vi "LuaVIEW Preprocessor.vi"(0 "path":path, 1 "parent index":i32, 5 "task info in":T2 {"handle mask" format="%.0b"; "allow mask" format="%.0b"; "signal flags" format="%.0b"}, 7 "script":string, 9 "main path valid?":bool, 11 "error in (no error)":errorcluster, 12 "main script?":bool, 13 "swap? (false)":bool) -> (4 "import paths":path[](array[path]), 6 "task info out":T2 {"handle mask" format="%.0b"; "allow mask" format="%.0b"; "signal flags" format="%.0b"}, 8 "script info":T1, 15 "error out":errorcluster)   [LabVIEW 2012]
doc: "Extract task configuration keywords from a script and configure the task state."
uses:
  typedefs/clusters/LuaVIEW Task Info.ctl
  typedefs/t_LuaVIEW Task Modes.ctl
  typedefs/t_LuaVIEW Reference.ctl
  typedefs/clusters/LuaVIEW Script Info.ctl
  typedefs/t_LuaVIEW Task List Methods.ctl
  typedefs/et_LuaVIEW CIN Actions.ctl
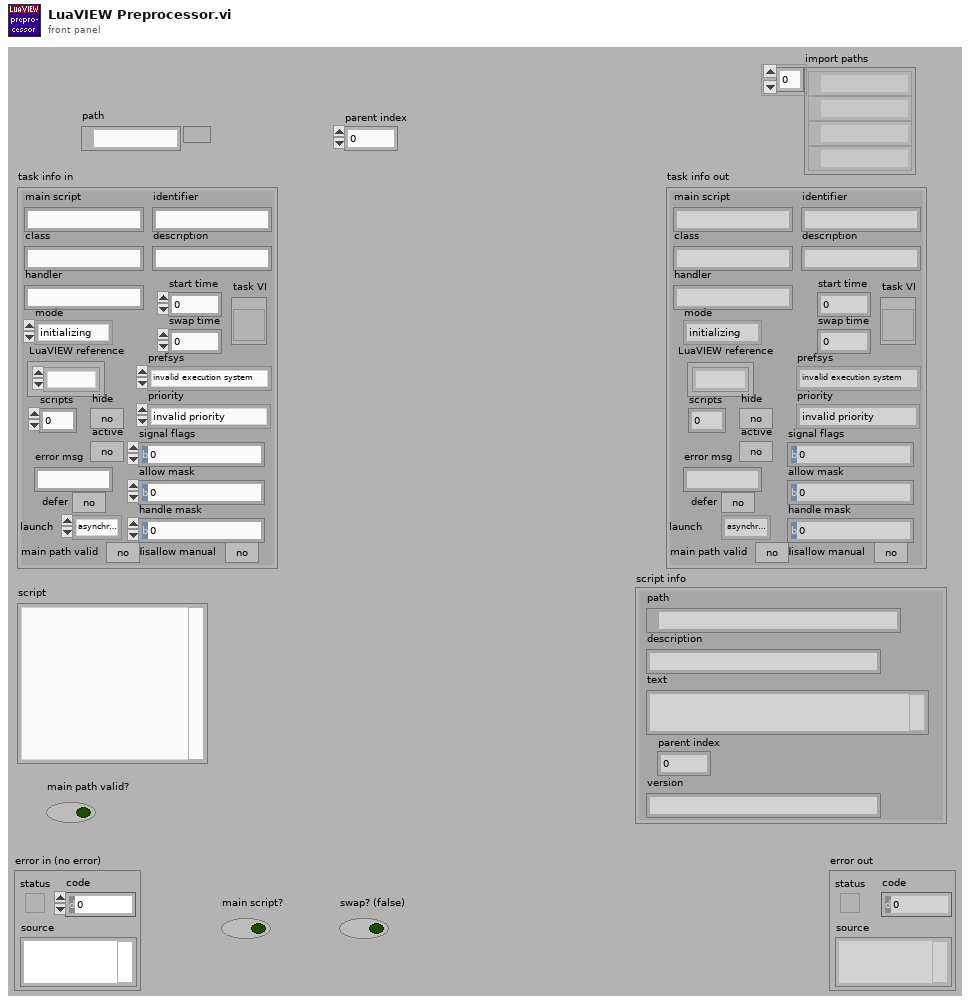
[diagram p1: front panel]
types:
  T1 = typedef "LuaVIEW Script Info.ctl" = cluster{"path":path, "description":string, "text":string, "parent index":i32, "version":string}
  T2 = typedef "LuaVIEW Task Info.ctl" = cluster{"main script":string, "identifier":string, "class":string, "description":string, "mode":T3, "handler":string, "LuaVIEW reference":T4, "scripts":i32, "hide":bool, "active":bool, "error msg":string, "defer":bool, "launch":enum16{"asynchronous", "manual", "synchronous"}, "main path valid":bool, "start time":dbl, "swap time":dbl, "task VI":refnum<vi>, "prefsys":enum32{"invalid execution system", "user interface", "standard", "instrument i/o", "data acquisition", "other 1", "other 2", "same as caller"}, "priority":enum32{"invalid priority", "background priority", "normal priority", "above normal priority", "high priority", "time critical priority", "subroutine"}, "signal flags":u32, "allow mask":u32, "handle mask":u32, "disallow manual":bool}
  T3 = typedef "t_LuaVIEW Task Modes.ctl" = enum16{"initializing", "running", "executing", "paused", "error", "swapping"}
  T4 = typedef "t_LuaVIEW Reference.ctl" = refnum<k1>
  T5 = typedef "t_LuaVIEW Task List Methods.ctl" = enum16{"clear list", "add", "test", "remove", "get ref", "get task info", "get list", "get script info", "ongoing?", "resume", "pause", "stop", "confirm", "message"}
  T6 = typedef "et_LuaVIEW CIN Actions.ctl" = enum16{"checksynopsis", "_open", "_registerpublic", "_registerexport", "__never_an_error_result_ns", "luaversion", "cinversion", "_totals", "_taskcount", "pathological", "_unregnextpublic", "registryusecount", "__per_state_actions", "regsetprivate", "regsetindex", "regsetmodule", "_revokeexports", "_usepublic", "prepare", "compile", "execute", "call", "unregstaterefs", "_close", "pullboolean", "pullnumber", "pullI8", "pullU8", "pullI16", "pullU16", "pullI32", "pullU32", "pullobject", "pullrefnum", "pullstring", "pullflat", "pushflat", "pushobject", "getattribute", "setattribute", "stacktostring", "_startyieldtest", "_endyieldtest", "_pollprintbuffer", "__never_an_error_result_ps", "_pollexport", "setclone", "forcecleanup", "gettop", "clearstack", "insert", "pushboolean", "pushnumber", "pushrefnum", "pushstring", "pushnil", "pushvalue", "gettaskref", "settaskref"}
  T7 = cluster{"line":i32, "keyword":string, "value":string}[]
  T8 = cluster{"line":i32, "keyword":string, "value":string}
  T9 = enum32{"invalid execution system", "user interface", "standard", "instrument i/o", "data acquisition", "other 1", "other 2", "same as caller"}
  T10 = enum32{"invalid priority", "background priority", "normal priority", "above normal priority", "high priority", "time critical priority", "subroutine"}
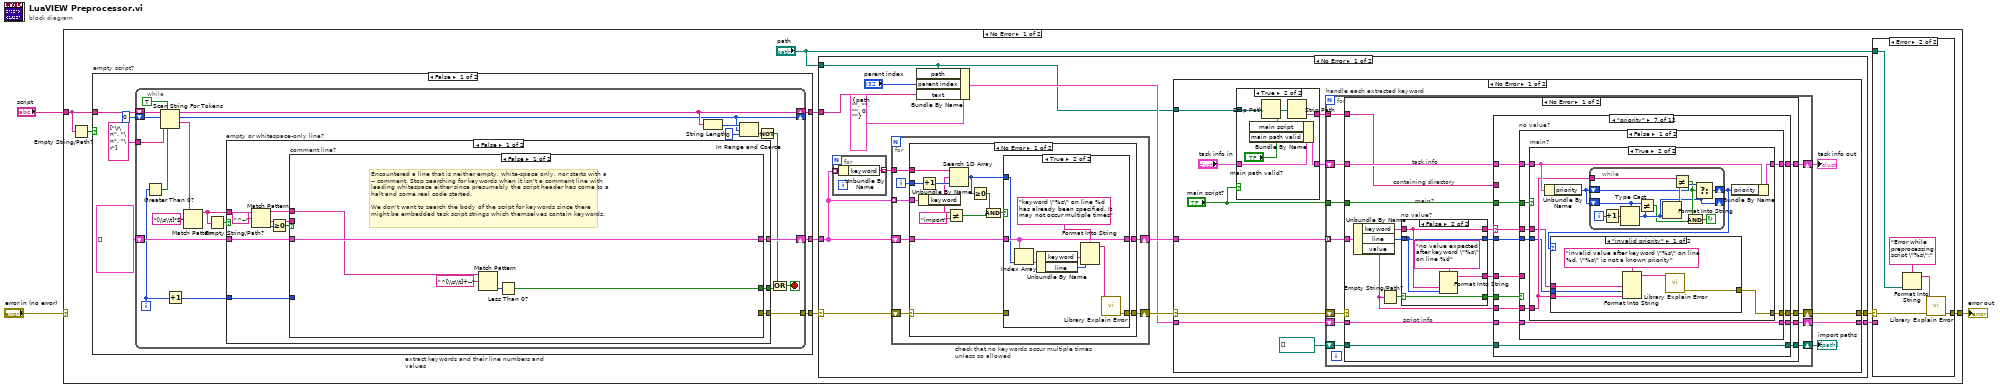
[diagram p0: block diagram]
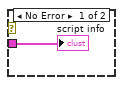
[diagram p2: hidden frame]
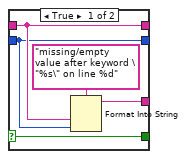
[diagram p4: hidden frame]
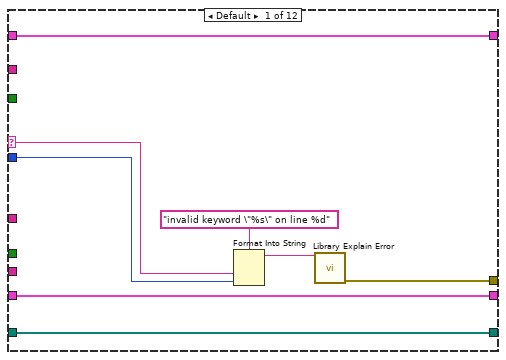
[diagram p5: hidden frame]
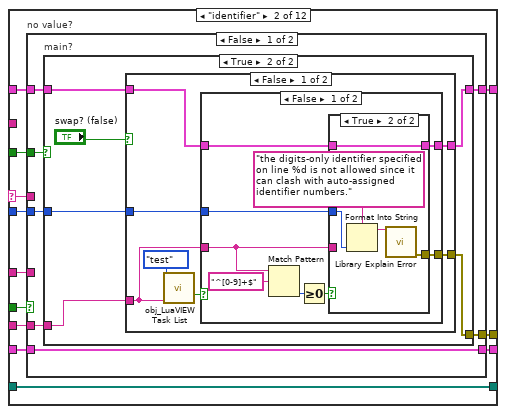
[diagram p6: hidden frame]
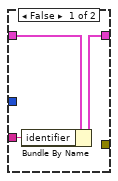
[diagram p8: hidden frame]
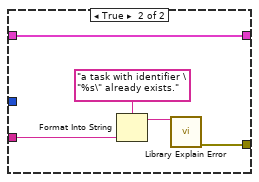
[diagram p9: hidden frame]
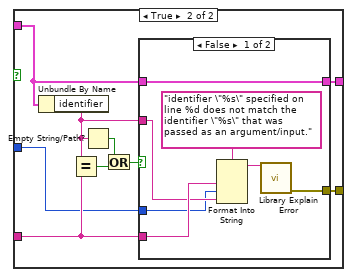
[diagram p10: hidden frame]
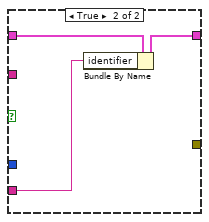
[diagram p11: hidden frame]
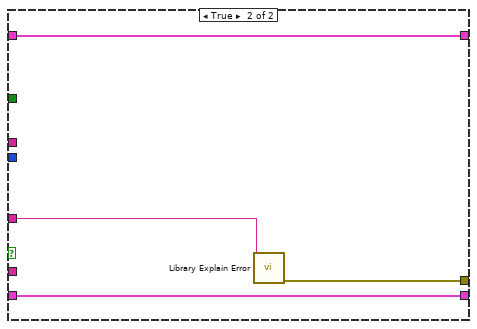
[diagram p12: hidden frame]
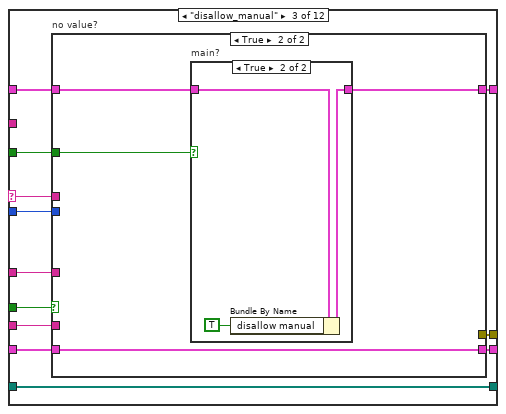
[diagram p13: hidden frame]
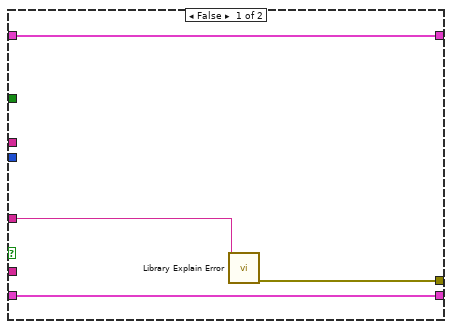
[diagram p14: hidden frame]
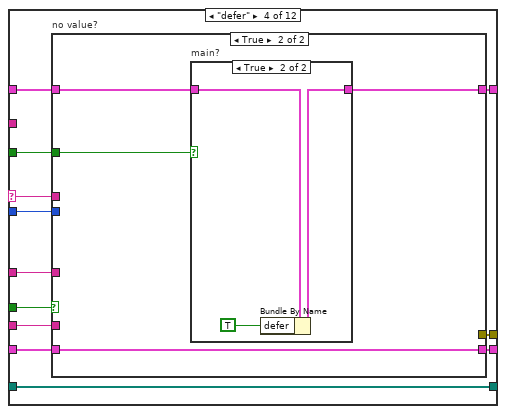
[diagram p16: hidden frame]
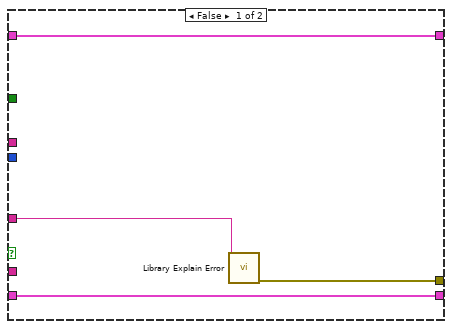
[diagram p17: hidden frame]
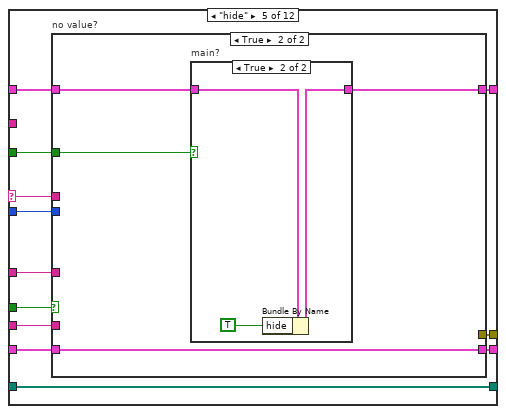
[diagram p19: hidden frame]
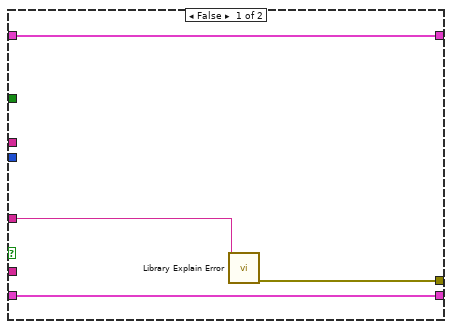
[diagram p20: hidden frame]
diagram:
  n1 = case shown="No Error" "error in (no error)" {
    selector: "error in (no error)" -> [_ w646]
    tunnel: "script" -> [w11 _]
    tunnel: [w5 w646] -> w1
    frame No Error {
      n2 = Empty String/Path?(string/path=w11) -> (empty?=w12:bool)
      n3 = case "empty script?" shown="False" w12 {
        tunnel: w11 -> [w539 w643]
        tunnel: [w537 w644] -> w10
        tunnel: [w536 w643] -> w9
        tunnel: [w535 _] -> w8
        frame False {
          n4 = while "extract keywords and their line numbers and values" {
            shift-right: [w547] -> w536
            shift-left: w539 -> [w563]
            tunnel: string[] ["\r\n", "\n", "\r"] ("delimiters (\\s,\\t,\\r,\\n)") -> [w562]
            shift-right: [w545] -> _
            shift-left: 0 ("offset past token") -> [w561]
            shift-right: [w548] -> w535
            shift-left: T7 [] -> [w554]
            tunnel: [w550] -> w537
            i -> [w551]
            stop <- w553 stop-if-true
            n5 = Greater Than 0?(x=w551) -> (x > 0?=w560:bool)
            n6 = Scan String For Tokens(4:w560, 5:TRUE ("allow empty tokens? (F)"), 6:w562, 8:w561, 9:w563) -> (1:w558:string, 2:w545:i32, 3:w547:string)  [unwired: 1 in, 1 out]
            n7 = Increment(x=w551) -> (x+1=w549:i32)
            n8 = Match Pattern(string=w558, regular expression="[\\s\\t]*$") -> (before substring=w556:string)  [unwired: 1 in, 3 out]
            n9 = Empty String/Path?(string/path=w556) -> (empty?=w555:bool)
            n10 = case "empty or whitespace-only line?" shown="False" w555 {
              tunnel: w556 -> [w573 _]
              tunnel: [w569 _] -> w552
              tunnel: w554 -> [w567 w642]
              tunnel: [w568 _] -> w550
              tunnel: w549 -> [w566 _]
              tunnel: [w565 w642] -> w548
              frame False {
                n11 = Match Pattern(string=w573, regular expression="^--") -> (before substring=w564:string, after substring=w570:string, offset past match=w572:i32)  [unwired: 1 in, 1 out]
                n12 = Greater Or Equal To 0?(x=w572) -> (x >= 0?=w571:bool)
                n13 = case "comment line?" shown="False" w571 {
                  tunnel: w570 -> [_ w580]
                  tunnel: [w576 w583] -> w569
                  tunnel: [_ w584] -> w568
                  tunnel: w567 -> [w579 w582]
                  tunnel: w566 -> [_ w585]
                  tunnel: [w579 w581] -> w565
                  tunnel: w564 -> [w575 _]
                  frame False {
                    # "Encountered a line that is neither empty, white-space only, nor starts with a -- comment. Stop searching for keywords when it isn't a comment line with leading whitespace either since presumably the script header has come to a halt and some real code started.\n\nWe don't want to search the body of the script for keywords since there might be embedded task script strings which themselves contain keywords."
                    n14 = Match Pattern(string=w575, regular expression="^[\\s\\t]+--") -> (offset past match=w577:i32)  [unwired: 1 in, 3 out]
                    n15 = Less Than 0?(x=w577) -> (x < 0?=w576:bool)
                  }
                  frame True {
                    n16 = Match Pattern(string=w580, regular expression="^#[a-z_]+") -> (match substring=w587:string, after substring=w588:string, offset past match=w592:i32)  [unwired: 1 in, 1 out]
                    n17 = Index Array(array=w582, index=-1) -> (element=w586:T8)
                    n18 = Greater Or Equal To 0?(x=w592) -> (x >= 0?=w590:bool)
                    n19 = case "looks like a keyword?" shown="True" w590 {
                      tunnel: w588 -> [_ w601]
                      tunnel: w587 -> [_ w606]
                      tunnel: w586 -> [_ w605]
                      tunnel: w585 -> [_ w604]
                      tunnel: [_ w594] -> w584
                      tunnel: [_ w595] -> w583
                      tunnel: w582 -> [w593 w598]
                      tunnel: [w593 w596] -> w581
                      frame False {
                      }
                      frame True {
                        n20 = String Subset(string=w606, offset (0)=1) -> (substring=w603:string)  [unwired: 1 in]
                        n21 = Bundle By Name(cluster=w605, "keyword"=w603, "line"=w604) -> (w599:T8)
                        n22 = Match Pattern(string=w601, regular expression="^[\\s\\t]*") -> (after substring=w597:string)  [unwired: 1 in, 3 out]
                        n23 = Empty String/Path?(string/path=w597) -> (empty?=w600:bool)
                        n24 = case "no trailing value?" shown="False" w600 {
                          tunnel: w599 -> [w613 w640]
                          tunnel: w598 -> [w614 w641]
                          tunnel: w597 -> [w625 _]
                          tunnel: [w612 w639] -> w596
                          tunnel: [w610 _] -> w595
                          tunnel: [w611 _] -> w594
                          frame False {
                            n25 = Search/Split String(string=w625, offset (0)=1) -> (substring before match=w619:string, match + rest of string=w622:string)  [unwired: 1 in, 1 out]
                            n26 = Equal?(x="\"" ("y"), y=w619) -> (x = y?=w617:bool)
                            n27 = String Length(string=w622) -> (length=w623:i32)
                            n28 = Decrement(x=w623) -> (x-1=w621:i32)
                            n29 = Search/Split String(string=w622, offset (0)=w621) -> (substring before match=w608:string, match + rest of string=w609:string)  [unwired: 1 in, 1 out]
                            n30 = Equal?(x="\"" ("y"), y=w609) -> (x = y?=w616:bool)
                            n31 = And(x=w617, y=w616) -> (x .and. y?=w615:bool)
                            n32 = case "proper double-quote delimited value?" shown="False" w615 {
                              tunnel: w614 -> [w633 w638]
                              tunnel: w613 -> [w632 w637]
                              tunnel: [w633 w635] -> w612
                              tunnel: [w631 _] -> w611
                              tunnel: [TRUE _] -> w610
                              tunnel: w608 -> [_ w634]
                              frame False {
                                n33 = Unbundle By Name(w632) -> ("keyword"=w628:string, "line"=w627:i32)
                                n34 = Format Into String(format string="value for keyword \"%s\" on line %d should be enclosed in double quotes.", w628, w627) -> (resulting string=w629:string)  [unwired: 2 in, 1 out]
                                n35 = call "Library Explain Error.vi"("explanation prefix (none)"=w629) -> ("explained error"=w631:errorcluster)  [unwired: 14 in]
                              }
                              frame True {
                                n36 = Bundle By Name(cluster=w637, "value"=w634) -> (w636:T8)
                                n37 = Build Array (concatenate)(w638, w636) -> (w635:T7)
                              }
                            }
                          }
                          frame True {
                            n38 = Build Array (concatenate)(w641, w640) -> (w639:T7)
                          }
                        }
                      }
                    }
                  }
                }
              }
              frame True {
              }
            }
            n39 = String Length(string=w547) -> (length=w546:i32)
            n40 = In Range and Coerce(upper limit=w546, x=w545, lower limit=0) -> (In Range?=w543:bool)  [unwired: 1 out]
            n41 = Not(x=w543) -> (.not. x?=w542:bool)
            n42 = Or(x=w542, y=w552) -> (x .or. y?=w553:bool)
          }
        }
        frame True {
          n43 = call "Library Explain Error.vi"("explanation prefix (none)"="script is empty") -> ("explained error"=w644:errorcluster)  [unwired: 14 in]
        }
      }
      n44 = case shown="No Error" w10 {
        selector: w10 -> [w30 w534]
        tunnel: w9 -> [w24 _]
        tunnel: w8 -> [w28 _]
        tunnel: "path" -> [w19 _]
        tunnel: [w21 _] -> w7
        tunnel: [w20 w534] -> w6
        frame No Error {
          n45 = for {
            tunnel: w28 -> [w533] mode=indexing
            tunnel: [w532] -> w29 mode=indexing
            n46 = Unbundle By Name(w533) -> ("keyword"=w532:string)
          }
          n47 = for "check that no keywords occur multiple times unless so allowed" {
            tunnel: w28 -> [w505] mode=indexing
            shift-right: [w499] -> w27
            shift-left: w30 -> [w503]
            tunnel: w29 -> [w502]
            shift-right: [w500] -> w26
            shift-left: w28 -> [w501]
            i -> [w504]
            n48 = case shown="No Error" w503 {
              selector: w503 -> [w506 w531]
              tunnel: w502 -> [w519 _]
              tunnel: w505 -> [w518 _]
              tunnel: w504 -> [w517 _]
              tunnel: w501 -> [w509 w530]
              tunnel: [w508 w530] -> w500
              tunnel: [w507 w531] -> w499
              frame No Error {
                n49 = Unbundle By Name(w518) -> ("keyword"=w515:string)
                n50 = Increment(x=w517) -> (x+1=w516:i32)
                n51 = Not Equal?(x=w515, y="import") -> (x != y?=w512:bool)
                n52 = Search 1D Array(1D array=w519, element=w515, start index (0)=w516) -> (index of element=w510:i32)
                n53 = Greater Or Equal To 0?(x=w510) -> (x >= 0?=w513:bool)
                n54 = And(x=w513, y=w512) -> (x .and. y?=w511:bool)
                n55 = case shown="True" w511 {
                  tunnel: w510 -> [_ w528]
                  tunnel: w509 -> [w520 w529]
                  tunnel: [w520 w529] -> w508
                  tunnel: [w521 w524] -> w507
                  tunnel: w506 -> [w521 _]
                  frame False {
                  }
                  frame True {
                    n56 = Index Array(array=w529, index=w528) -> (element=w527:T8)
                    n57 = Unbundle By Name(w527) -> ("keyword"=w526:string, "line"=w522:i32)
                    n58 = Format Into String(format string="keyword \"%s\" on line %d  has already been specified. It may not occur multiple times", w526, w522) -> (resulting string=w523:string)  [unwired: 2 in, 1 out]
                    n59 = call "Library Explain Error.vi"("explanation prefix (none)"=w523) -> ("explained error"=w524:errorcluster)  [unwired: 14 in]
                  }
                }
              }
              frame Error {
              }
            }
          }
          n60 = Bundle By Name(cluster=T1 {"path"=path "", "description"="", "text"="", "parent index"=0, "version"=""} ("script info"), "path"=w19, "parent index"="parent index", "text"=w24) -> (w23:T1)
          n61 = case shown="No Error" w27 {
            selector: w27 -> [w43 w498]
            tunnel: w26 -> [w42 _]
            tunnel: w19 -> [w39 _]
            tunnel: w23 -> [w38 w497]
            tunnel: [w33 w497] -> w21
            tunnel: [w32 w498] -> w20
            frame No Error {
              n62 = case shown="True" "main script?" {
                tunnel: w39 -> [_ w48]
                tunnel: [w44 w49] -> w41
                tunnel: "task info in" -> [w44 w47]
                tunnel: [_ w45] -> w31
                frame False {
                }
                frame True {
                  n63 = Strip Path(path=w48) -> (stripped path=w46:path, name=w51:string)
                  n64 = Bundle By Name(cluster=w47, "main script"=w51, "main path valid"="main path valid?") -> (w49:T2)
                  n65 = Strip Path(path=w46) -> (name=w45:string)  [unwired: 1 out]
                }
              }
              n66 = for "handle each extracted keyword" {
                shift-right: [w57] -> w32
                shift-left: w43 -> [w58]
                tunnel: w42 -> [w59] mode=indexing
                shift-right: [w61] -> w37
                shift-left: w41 -> [w62]
                tunnel: "main script?" -> [w60]
                shift-right: [w53] -> w34
                shift-left: path[] [] ("import paths") -> [w56]
                shift-right: [w54] -> w33
                shift-left: w38 -> [w55]
                tunnel: w31 -> [w52]
                n67 = case shown="No Error" w58 {
                  selector: w58 -> [_ w495]
                  tunnel: w62 -> [w80 w496]
                  tunnel: [w79 w496] -> w61
                  tunnel: w60 -> [w78 _]
                  tunnel: w59 -> [w77 _]
                  tunnel: [w68 w495] -> w57
                  tunnel: w56 -> [w67 w493]
                  tunnel: w55 -> [w66 w494]
                  tunnel: [w65 w494] -> w54
                  tunnel: [w64 w493] -> w53
                  tunnel: w52 -> [w63 _]
                  frame No Error {
                    # "containing directory"
                    # "main?"
                    # "task info"
                    # "script info"
                    n68 = Unbundle By Name(w77) -> ("keyword"=w76:string, "line"=w75:i32, "value"=w72:string)
                    n69 = Empty String/Path?(string/path=w72) -> (empty?=w73:bool)
                    n70 = case "no value?" shown="False" w73 {
                      selector: w73 -> [w81 w86]
                      tunnel: w76 -> [w83 w88]
                      tunnel: w75 -> [w82 w87]
                      tunnel: [w84 w89] -> w69
                      tunnel: [w83 w88] -> w71
                      tunnel: [w82 w87] -> w74
                      tunnel: [w81 w86] -> w70
                      frame True {
                        n71 = Format Into String(format string="missing/empty value after keyword \"%s\" on line %d", w83, w82) -> (resulting string=w84:string)  [unwired: 2 in, 1 out]
                      }
                      frame False {
                        n72 = Format Into String(format string="no value expected after keyword \"%s\" on line %d", w88, w87) -> (resulting string=w89:string)  [unwired: 2 in, 1 out]
                      }
                    }
                    n73 = case shown="\"priority\"" w71 {
                      selector: w71 -> [w98 w104 w181 w205 w229 w253 w303 w354 w384 _ w452 w473]
                      tunnel: w74 -> [w97 w103 w180 w204 w228 w252 w302 w353 w383 w409 w451 w472]
                      tunnel: [w94 w108 w185 w209 w233 w257 w307 w358 w388 w413 w456 w477] -> w68
                      tunnel: w80 -> [w93 w109 w186 w210 w234 w258 w308 w359 w389 w414 w457 w478]
                      tunnel: [w93 w102 w179 w203 w227 w251 w301 w352 w382 w408 w450 w471] -> w79
                      tunnel: w78 -> [_ w110 w187 w211 w235 w259 w309 w360 w390 w415 w458 w479]
                      tunnel: w72 -> [_ w105 w182 w206 w230 w254 w304 w355 w385 w410 w453 w474]
                      tunnel: w70 -> [_ w107 w184 w208 w232 w256 w306 w357 w387 w412 w455 w476]
                      tunnel: w69 -> [_ w106 w183 w207 w231 w255 w305 w356 w386 w411 w454 w475]
                      tunnel: w67 -> [w91 w99 w176 w200 w224 w248 w298 w349 w379 w405 w447 w468]
                      tunnel: w66 -> [w92 w101 w178 w202 w226 w250 w300 w351 w381 w407 w449 w470]
                      tunnel: [w92 w100 w177 w201 w225 w249 w299 w350 w380 w406 w448 w469] -> w65
                      tunnel: [w91 w99 w176 w200 w224 w248 w298 w349 w379 w405 w447 w467] -> w64
                      tunnel: w63 -> [_ _ _ _ _ _ _ w348 _ _ _ _]
                      frame Default {
                        n74 = Format Into String(format string="invalid keyword \"%s\" on line %d", w98, w97) -> (resulting string=w95:string)  [unwired: 2 in, 1 out]
                        n75 = call "Library Explain Error.vi"("explanation prefix (none)"=w95) -> ("explained error"=w94:errorcluster)  [unwired: 14 in]
                      }
                      frame "identifier" {
                        n76 = case "no value?" shown="False" w107 {
                          tunnel: w110 -> [w114 _]
                          tunnel: w103 -> [w111 _]
                          tunnel: w104 -> [_ _]
                          tunnel: w109 -> [w116 w173]
                          tunnel: [w112 w175] -> w108
                          tunnel: w106 -> [_ w174]
                          tunnel: w105 -> [w117 _]
                          tunnel: [w115 w173] -> w102
                          tunnel: [w113 w172] -> w100
                          tunnel: w101 -> [w113 w172]
                          frame False {
                            n77 = case "main?" shown="True" w114 {
                              tunnel: w117 -> [_ w121]
                              tunnel: w116 -> [w118 w124]
                              tunnel: [w118 w123] -> w115
                              tunnel: [_ w122] -> w112
                              tunnel: w111 -> [_ w119]
                              frame False {
                              }
                              frame True {
                                n78 = case shown="False" "swap? (false)" {
                                tunnel: w124 -> [w131 w157]
                                tunnel: [w130 w158] -> w123
                                tunnel: [w129 w155] -> w122
                                tunnel: w121 -> [w126 w156]
                                tunnel: w119 -> [w125 w153]
                                frame False {
                                n79 = call "obj_LuaVIEW Task List.vi"("method"=t_LuaVIEW_Task_List_Methods."test", "task identifier"=w126) -> ("set/ongoing"=w127:bool)  [unwired: 8 in, 5 out]
                                n80 = case shown="False" w127 {
                                tunnel: [w137 w152] -> w129
                                tunnel: w126 -> [w135 w150]
                                tunnel: w131 -> [w139 w148]
                                tunnel: [w138 w148] -> w130
                                tunnel: w125 -> [w132 _]
                                frame False {
                                n81 = Match Pattern(string=w135, regular expression="^[0-9]+$") -> (offset past match=w134:i32)  [unwired: 1 in, 3 out]
                                n82 = Greater Or Equal To 0?(x=w134) -> (x >= 0?=w133:bool)
                                n83 = case shown="True" w133 {
                                tunnel: w135 -> [w142 _]
                                tunnel: w139 -> [w141 w147]
                                tunnel: [w140 w147] -> w138
                                tunnel: [_ w146] -> w137
                                tunnel: w132 -> [_ w145]
                                frame False {
                                n84 = Bundle By Name(cluster=w141, "identifier"=w142) -> (w140:T2)
                                }
                                frame True {
                                n85 = Format Into String(format string="the digits-only identifier specified on line %d is not allowed since it can clash with auto-assigned identifier numbers.", w145) -> (resulting string=w144:string)  [unwired: 2 in, 1 out]
                                n86 = call "Library Explain Error.vi"("explanation prefix (none)"=w144) -> ("explained error"=w146:errorcluster)  [unwired: 14 in]
                                }
                                }
                                }
                                frame True {
                                n87 = Format Into String(format string="a task with identifier \"%s\" already exists.", w150) -> (resulting string=w151:string)  [unwired: 2 in, 1 out]
                                n88 = call "Library Explain Error.vi"("explanation prefix (none)"=w151) -> ("explained error"=w152:errorcluster)  [unwired: 14 in]
                                }
                                }
                                }
                                frame True {
                                n89 = Unbundle By Name(w157) -> ("identifier"=w154:string)
                                n90 = Equal?(x=w154, y=w156) -> (x = y?=w161:bool)
                                n91 = Empty String/Path?(string/path=w154) -> (empty?=w160:bool)
                                n92 = Or(x=w160, y=w161) -> (x .or. y?=w159:bool)
                                n93 = case shown="False" w159 {
                                tunnel: [w165 w171] -> w158
                                tunnel: w157 -> [w165 w170]
                                tunnel: w156 -> [w164 w169]
                                tunnel: [w166 _] -> w155
                                tunnel: w154 -> [w163 _]
                                tunnel: w153 -> [w162 _]
                                frame False {
                                n94 = Format Into String(format string="identifier \"%s\" specified on line %d does not match the  identifier \"%s\" that was passed as an argument/input.", w164, w162, w163) -> (resulting string=w168:string)  [unwired: 2 in, 1 out]
                                n95 = call "Library Explain Error.vi"("explanation prefix (none)"=w168) -> ("explained error"=w166:errorcluster)  [unwired: 14 in]
                                }
                                frame True {
                                n96 = Bundle By Name(cluster=w170, "identifier"=w169) -> (w171:T2)
                                }
                                }
                                }
                                }
                              }
                            }
                          }
                          frame True {
                            n97 = call "Library Explain Error.vi"("explanation prefix (none)"=w174) -> ("explained error"=w175:errorcluster)  [unwired: 14 in]
                          }
                        }
                      }
                      frame "disallow_manual" {
                        n98 = case "no value?" shown="True" w184 {
                          tunnel: w187 -> [_ w193]
                          tunnel: w180 -> [_ _]
                          tunnel: w181 -> [_ _]
                          tunnel: w186 -> [w189 w195]
                          tunnel: [w191 _] -> w185
                          tunnel: w183 -> [w190 _]
                          tunnel: w182 -> [_ _]
                          tunnel: [w189 w194] -> w179
                          tunnel: [w188 w192] -> w177
                          tunnel: w178 -> [w188 w192]
                          frame False {
                            n99 = call "Library Explain Error.vi"("explanation prefix (none)"=w190) -> ("explained error"=w191:errorcluster)  [unwired: 14 in]
                          }
                          frame True {
                            n100 = case "main?" shown="True" w193 {
                              tunnel: w195 -> [w196 w199]
                              tunnel: [w196 w198] -> w194
                              frame False {
                              }
                              frame True {
                                n101 = Bundle By Name(cluster=w199, "disallow manual"=TRUE) -> (w198:T2)
                              }
                            }
                          }
                        }
                      }
                      frame "defer" {
                        n102 = case "no value?" shown="True" w208 {
                          tunnel: w211 -> [_ w217]
                          tunnel: w204 -> [_ _]
                          tunnel: w205 -> [_ _]
                          tunnel: w210 -> [w213 w219]
                          tunnel: [w215 _] -> w209
                          tunnel: w207 -> [w214 _]
                          tunnel: w206 -> [_ _]
                          tunnel: [w213 w218] -> w203
                          tunnel: [w212 w216] -> w201
                          tunnel: w202 -> [w212 w216]
                          frame False {
                            n103 = call "Library Explain Error.vi"("explanation prefix (none)"=w214) -> ("explained error"=w215:errorcluster)  [unwired: 14 in]
                          }
                          frame True {
                            n104 = case "main?" shown="True" w217 {
                              tunnel: w219 -> [w220 w223]
                              tunnel: [w220 w222] -> w218
                              frame False {
                              }
                              frame True {
                                n105 = Bundle By Name(cluster=w223, "defer"=TRUE ("disallow manual")) -> (w222:T2)
                              }
                            }
                          }
                        }
                      }
                      frame "hide" {
                        n106 = case "no value?" shown="True" w232 {
                          tunnel: w235 -> [_ w241]
                          tunnel: w228 -> [_ _]
                          tunnel: w229 -> [_ _]
                          tunnel: w234 -> [w237 w243]
                          tunnel: [w239 _] -> w233
                          tunnel: w231 -> [w238 _]
                          tunnel: w230 -> [_ _]
                          tunnel: [w237 w242] -> w227
                          tunnel: [w236 w240] -> w225
                          tunnel: w226 -> [w236 w240]
                          frame False {
                            n107 = call "Library Explain Error.vi"("explanation prefix (none)"=w238) -> ("explained error"=w239:errorcluster)  [unwired: 14 in]
                          }
                          frame True {
                            n108 = case "main?" shown="True" w241 {
                              tunnel: w243 -> [w244 w247]
                              tunnel: [w244 w246] -> w242
                              frame False {
                              }
                              frame True {
                                n109 = Bundle By Name(cluster=w247, "hide"=TRUE ("disallow manual")) -> (w246:T2)
                              }
                            }
                          }
                        }
                      }
                      frame "prefsys" {
                        n110 = case "no value?" shown="False" w256 {
                          tunnel: w259 -> [w265 _]
                          tunnel: w252 -> [w262 _]
                          tunnel: w253 -> [w260 _]
                          tunnel: w258 -> [w267 w295]
                          tunnel: [w261 w297] -> w257
                          tunnel: w255 -> [_ w296]
                          tunnel: w254 -> [w263 _]
                          tunnel: [w266 w295] -> w251
                          tunnel: [w264 w294] -> w249
                          tunnel: w250 -> [w264 w294]
                          frame False {
                            n111 = case "main?" shown="True" w265 {
                              tunnel: w267 -> [w268 w275]
                              tunnel: [w268 w276] -> w266
                              tunnel: w263 -> [_ w272]
                              tunnel: w260 -> [_ w271]
                              tunnel: w262 -> [_ w270]
                              tunnel: [_ w269] -> w261
                              frame False {
                              }
                              frame True {
                                n112 = Unbundle By Name(w275) -> ("prefsys"=w274:T9)
                                n113 = while {
                                shift-right: [w289] -> w273
                                shift-left: w274 -> [w288]
                                shift-right: [w285] -> _
                                shift-left: w274 -> [w292]
                                tunnel: w272 -> [w291]
                                i -> [w293]
                                stop <- w286 continue-if-true
                                n114 = Increment(x=w293) -> (x+1=w283:i32)
                                n115 = Type Cast(type=w292, x=w283) -> (*(type *) &x=w285:T9)
                                n116 = Not Equal?(x=w292, y=w285) -> (x != y?=w284:bool)
                                n117 = Format Into String(w285) -> (resulting string=w290:string)  [unwired: 3 in, 1 out]
                                n118 = Not Equal?(x=w291, y=w290) -> (x != y?=w287:bool)
                                n119 = And(x=w287, y=w284) -> (x .and. y?=w286:bool)
                                n120 = Select(t=w288, s=w287, f=w285) -> (s? t:f=w289:T9)
                                }
                                n121 = case shown="\"invalid execution system\"" w273 {
                                tunnel: w272 -> [w281 _]
                                tunnel: w271 -> [w280 _]
                                tunnel: w270 -> [w279 _]
                                tunnel: [w277 _] -> w269
                                frame "invalid execution system" {
                                n122 = Format Into String(format string="invalid value after keyword \"%s\" on line %d, \"%s\" is not a known execution system", w280, w279, w281) -> (resulting string=w278:string)  [unwired: 2 in, 1 out]
                                n123 = call "Library Explain Error.vi"("explanation prefix (none)"=w278) -> ("explained error"=w277:errorcluster)  [unwired: 14 in]
                                }
                                frame Default {
                                }
                                }
                                n124 = Bundle By Name(cluster=w275, "prefsys"=w273) -> (w276:T2)
                              }
                            }
                          }
                          frame True {
                            n125 = call "Library Explain Error.vi"("explanation prefix (none)"=w296) -> ("explained error"=w297:errorcluster)  [unwired: 14 in]
                          }
                        }
                      }
                      frame "priority" {
                        n126 = case "no value?" shown="False" w306 {
                          tunnel: w309 -> [w315 _]
                          tunnel: w302 -> [w312 _]
                          tunnel: w303 -> [w310 _]
                          tunnel: w308 -> [w317 w345]
                          tunnel: [w311 w347] -> w307
                          tunnel: w305 -> [_ w346]
                          tunnel: w304 -> [w313 _]
                          tunnel: [w316 w345] -> w301
                          tunnel: [w314 w344] -> w299
                          tunnel: w300 -> [w314 w344]
                          frame False {
                            n127 = case "main?" shown="True" w315 {
                              tunnel: w317 -> [w318 w325]
                              tunnel: [w318 w326] -> w316
                              tunnel: w313 -> [_ w322]
                              tunnel: w310 -> [_ w321]
                              tunnel: w312 -> [_ w320]
                              tunnel: [_ w319] -> w311
                              frame False {
                              }
                              frame True {
                                n128 = Unbundle By Name(w325) -> ("priority"=w324:T10)
                                n129 = while {
                                shift-right: [w339] -> w323
                                shift-left: w324 -> [w338]
                                shift-right: [w335] -> _
                                shift-left: w324 -> [w342]
                                tunnel: w322 -> [w341]
                                i -> [w343]
                                stop <- w336 continue-if-true
                                n130 = Increment(x=w343) -> (x+1=w333:i32)
                                n131 = Type Cast(type=w342, x=w333) -> (*(type *) &x=w335:T10)
                                n132 = Not Equal?(x=w342, y=w335) -> (x != y?=w334:bool)
                                n133 = Format Into String(w335) -> (resulting string=w340:string)  [unwired: 3 in, 1 out]
                                n134 = Not Equal?(x=w341, y=w340) -> (x != y?=w337:bool)
                                n135 = And(x=w337, y=w334) -> (x .and. y?=w336:bool)
                                n136 = Select(t=w338, s=w337, f=w335) -> (s? t:f=w339:T10)
                                }
                                n137 = case shown="\"invalid priority\"" w323 {
                                tunnel: w322 -> [w331 _]
                                tunnel: w321 -> [w330 _]
                                tunnel: w320 -> [w329 _]
                                tunnel: [w327 _] -> w319
                                frame "invalid priority" {
                                n138 = Format Into String(format string="invalid value after keyword \"%s\" on line %d, \"%s\" is not a known priority", w330, w329, w331) -> (resulting string=w328:string)  [unwired: 2 in, 1 out]
                                n139 = call "Library Explain Error.vi"("explanation prefix (none)"=w328) -> ("explained error"=w327:errorcluster)  [unwired: 14 in]
                                }
                                frame Default {
                                }
                                }
                                n140 = Bundle By Name(cluster=w325, "priority"=w323) -> (w326:T2)
                              }
                            }
                          }
                          frame True {
                            n141 = call "Library Explain Error.vi"("explanation prefix (none)"=w346) -> ("explained error"=w347:errorcluster)  [unwired: 14 in]
                          }
                        }
                      }
                      frame "class" {
                        n142 = case "no value?" shown="False" w357 {
                          tunnel: w360 -> [w363 _]
                          tunnel: w353 -> [_ _]
                          tunnel: w354 -> [_ _]
                          tunnel: w359 -> [w365 w376]
                          tunnel: [_ w378] -> w358
                          tunnel: w356 -> [_ w377]
                          tunnel: w355 -> [w366 _]
                          tunnel: [w364 w376] -> w352
                          tunnel: [w362 w375] -> w350
                          tunnel: w351 -> [w362 w375]
                          tunnel: w348 -> [w361 _]
                          frame False {
                            n143 = case "main?" shown="True" w363 {
                              tunnel: w366 -> [_ w369]
                              tunnel: w365 -> [w367 w374]
                              tunnel: [w367 w373] -> w364
                              tunnel: w361 -> [_ w371]
                              frame False {
                              }
                              frame True {
                                n144 = Equal?(x="<dir>", y=w369) -> (x = y?=w370:bool)
                                n145 = Select(t=w371, s=w370, f=w369) -> (s? t:f=w372:string)
                                n146 = Bundle By Name(cluster=w374, "class"=w372) -> (w373:T2)
                              }
                            }
                          }
                          frame True {
                            n147 = call "Library Explain Error.vi"("explanation prefix (none)"=w377) -> ("explained error"=w378:errorcluster)  [unwired: 14 in]
                          }
                        }
                      }
                      frame "description" {
                        n148 = case "no value?" shown="False" w387 {
                          tunnel: w390 -> [w394 _]
                          tunnel: w383 -> [_ _]
                          tunnel: w384 -> [_ _]
                          tunnel: w389 -> [w396 w402]
                          tunnel: [_ w404] -> w388
                          tunnel: w386 -> [_ w403]
                          tunnel: w385 -> [w391 _]
                          tunnel: [w395 w402] -> w382
                          tunnel: [w392 w401] -> w380
                          tunnel: w381 -> [w393 w401]
                          frame False {
                            n149 = Bundle By Name(cluster=w393, "description"=w391) -> (w392:T1)
                            n150 = case "main?" shown="True" w394 {
                              tunnel: w391 -> [_ w400]
                              tunnel: w396 -> [w397 w399]
                              tunnel: [w397 w398] -> w395
                              frame False {
                              }
                              frame True {
                                n151 = Bundle By Name(cluster=w399, "description"=w400) -> (w398:T2)
                              }
                            }
                          }
                          frame True {
                            n152 = call "Library Explain Error.vi"("explanation prefix (none)"=w403) -> ("explained error"=w404:errorcluster)  [unwired: 14 in]
                          }
                        }
                      }
                      frame "handler" {
                        n153 = case "no value?" shown="False" w412 {
                          tunnel: w415 -> [w420 _]
                          tunnel: w409 -> [w417 _]
                          tunnel: w414 -> [w422 w444]
                          tunnel: [w416 w446] -> w413
                          tunnel: w411 -> [_ w445]
                          tunnel: w410 -> [w419 _]
                          tunnel: [w421 w444] -> w408
                          tunnel: [w418 w443] -> w406
                          tunnel: w407 -> [w418 w443]
                          frame False {
                            n154 = case "main?" shown="True" w420 {
                              tunnel: w419 -> [_ w428]
                              tunnel: w422 -> [w423 w427]
                              tunnel: [w423 w429] -> w421
                              tunnel: w417 -> [_ w425]
                              tunnel: [_ w424] -> w416
                              frame False {
                              }
                              frame True {
                                n155 = Unbundle By Name(w427) -> ("launch"=w426:enum16{"asynchronous", "manual", "synchronous"})
                                n156 = case shown="\"asynchronous\", \"manual\"" w426 {
                                tunnel: w427 -> [w430 w437]
                                tunnel: [w430 w436] -> w429
                                tunnel: w428 -> [_ w431]
                                tunnel: w425 -> [_ w433]
                                tunnel: [_ w432] -> w424
                                frame "synchronous" {
                                }
                                frame "asynchronous", "manual" {
                                n157 = call "obj_LuaVIEW Task List.vi"("method"=t_LuaVIEW_Task_List_Methods."test", "task identifier"=w431) -> ("set/ongoing"=w434:bool)  [unwired: 8 in, 5 out]
                                n158 = Bundle By Name(cluster=w437, "handler"=w431) -> (w436:T2)
                                n159 = case shown="False" w434 {
                                tunnel: w433 -> [w438 _]
                                tunnel: [w441 _] -> w432
                                tunnel: w431 -> [w439 _]
                                frame False {
                                n160 = Format Into String(format string="no handler task with identifier \"%s\" as specified on line %d exists", w439, w438) -> (resulting string=w442:string)  [unwired: 2 in, 1 out]
                                n161 = call "Library Explain Error.vi"("explanation prefix (none)"=w442) -> ("explained error"=w441:errorcluster)  [unwired: 14 in]
                                }
                                frame True {
                                }
                                }
                                }
                                }
                              }
                            }
                          }
                          frame True {
                            n162 = call "Library Explain Error.vi"("explanation prefix (none)"=w445) -> ("explained error"=w446:errorcluster)  [unwired: 14 in]
                          }
                        }
                      }
                      frame "version" {
                        n163 = case "no value?" shown="False" w455 {
                          tunnel: w458 -> [_ _]
                          tunnel: w451 -> [_ _]
                          tunnel: w452 -> [_ _]
                          tunnel: w457 -> [w459 w464]
                          tunnel: [_ w466] -> w456
                          tunnel: w454 -> [_ w465]
                          tunnel: w453 -> [w460 _]
                          tunnel: [w459 w464] -> w450
                          tunnel: [w461 w463] -> w448
                          tunnel: w449 -> [w462 w463]
                          frame False {
                            n164 = Bundle By Name(cluster=w462, "version"=w460) -> (w461:T1)
                          }
                          frame True {
                            n165 = call "Library Explain Error.vi"("explanation prefix (none)"=w465) -> ("explained error"=w466:errorcluster)  [unwired: 14 in]
                          }
                        }
                      }
                      frame "import" {
                        n166 = case "no value?" shown="False" w476 {
                          tunnel: w479 -> [_ _]
                          tunnel: w472 -> [_ _]
                          tunnel: w473 -> [_ _]
                          tunnel: w478 -> [w487 w490]
                          tunnel: [_ w492] -> w477
                          tunnel: w475 -> [_ w491]
                          tunnel: w474 -> [w483 _]
                          tunnel: [w487 w490] -> w471
                          tunnel: [w486 w489] -> w469
                          tunnel: w470 -> [w486 w489]
                          tunnel: w468 -> [w481 w488]
                          tunnel: [w480 w488] -> w467
                          frame False {
                            n167 = call "re_LuaVIEW CIN.vi"("action"=et_LuaVIEW_CIN_Actions."pathological", "string in"=w483) -> ("string out"=w485:string)  [unwired: 7 in, 6 out]
                            n168 = String To Path(string=w485) -> (path=w482:path)
                            n169 = Build Array (concatenate)(w481, w482) -> (w480:path[])
                          }
                          frame True {
                            n170 = call "Library Explain Error.vi"("explanation prefix (none)"=w491) -> ("explained error"=w492:errorcluster)  [unwired: 14 in]
                          }
                        }
                      }
                    }
                  }
                  frame Error {
                  }
                }
              }
              "task info out" <- w37
              "import paths" <- w34
            }
            frame Error {
            }
          }
        }
        frame Error {
        }
      }
      n171 = case shown="Error" w6 {
        selector: w6 -> [_ w18]
        tunnel: w7 -> [w13 _]
        tunnel: [_ w17] -> w5
        tunnel: "path" -> [_ w14]
        frame No Error {
          "script info" <- w13
        }
        frame Error {
          n172 = Format Into String(format string="Error while preprocessing script \"%s\":", w14) -> (resulting string=w15:string)  [unwired: 2 in, 1 out]
          n173 = call "Library Explain Error.vi"("explanation prefix (none)"=w15, "error in (no error)"=w18) -> ("explained error"=w17:errorcluster)  [unwired: 13 in]
        }
      }
    }
    frame Error {
    }
  }
  "error out" <- w1
